vi "_Parse ES Flatness Limit Check Result.vi"(8 "error in (no error)":errorcluster, 10 "Input String":string, 11 "VISA resource name":refnum<visa-resource-name>) -> (0 "error out":errorcluster, 1 "Result":T1 {"Out Of Tolerance" format="%^.3e"}, 2 "Reliability":i32, 3 "VISA resource name out":refnum<visa-resource-name>)   [LabVIEW 2015, in "Rohde&Schwarz CMXP NR FR2 Measurement.lvlib"]
uses:
  <instrlib>/Rohde&Schwarz CMXP NR FR2 Measurement/Rohde&Schwarz CMXP NR FR2 Measurement.lvlib
  <instrlib>/Rohde&Schwarz CMXP NR FR2 Measurement/Private/rsidr_core.llb/rsidr_core.lvlib
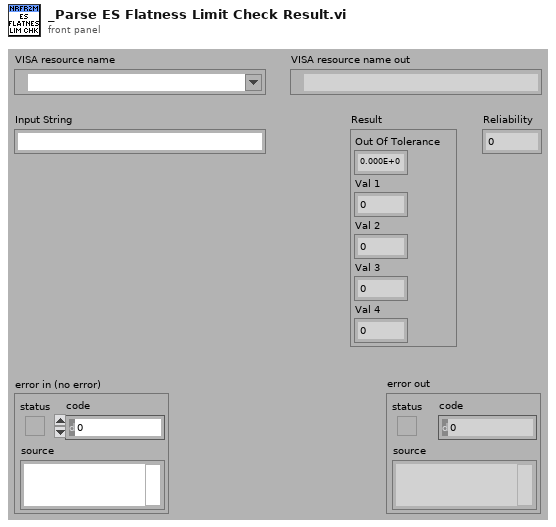
[diagram p1: front panel]
types:
  T1 = cluster{"Out Of Tolerance":dbl, "Val 1":i32, "Val 2":i32, "Val 3":i32, "Val 4":i32}
  T2 = cluster{"Out Of Tolerance":dbl, "Ripple 1":i32, "Ripple 2":i32, "Max R1 Min R2":i32, "Max R2 Min R1":i32}
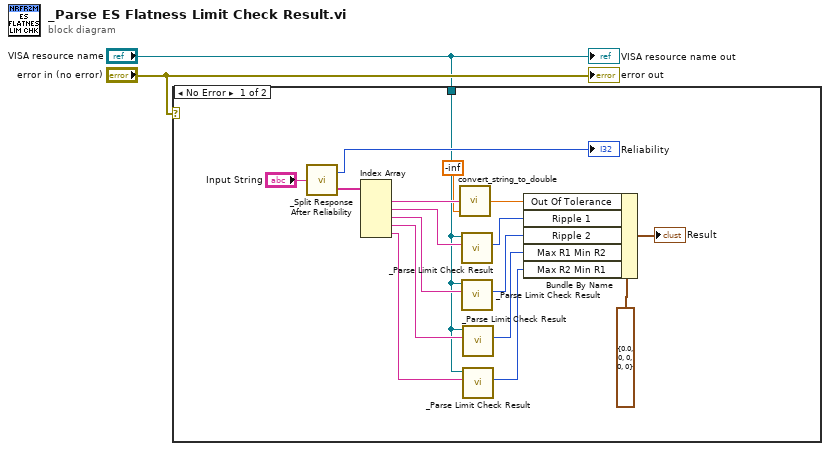
[diagram p0: block diagram]
diagram:
  n1 = case shown="No Error" "error in (no error)" {
    tunnel: "VISA resource name" -> [w3 _]
    frame No Error {
      n2 = call <instrlib>:"_Split Response After Reliability.vi"("Input String"="Input String") -> ("Response out"=w13:string[], "Reliability out"=→"Reliability":i32)
      n3 = Index Array(array=w13) -> (element #1=w12:string, element #2=w11:string, element #3=w10:string, element #4=w7:string, element #5=w8:string)  [unwired: 5 in]
      n4 = call <instrlib>:"convert_string_to_double.vi"("default (0)"=-inf, "String in"=w12) -> ("double value out"=w18:dbl)  [unwired: 3 in]
      n5 = call <instrlib>:"_Parse Limit Check Result.vi"("String Value In"=w11, "VISA resource name"=w3) -> ("Limit Check Value"=w17:i32)  [unwired: 7 in, 2 out]
      n6 = call <instrlib>:"_Parse Limit Check Result.vi"("String Value In"=w10, "VISA resource name"=w3) -> ("Limit Check Value"=w16:i32)  [unwired: 7 in, 2 out]
      n7 = call <instrlib>:"_Parse Limit Check Result.vi"("String Value In"=w7, "VISA resource name"=w3) -> ("Limit Check Value"=w5:i32)  [unwired: 7 in, 2 out]
      n8 = call <instrlib>:"_Parse Limit Check Result.vi"("String Value In"=w8, "VISA resource name"=w3) -> ("Limit Check Value"=w4:i32)  [unwired: 7 in, 2 out]
      n9 = Bundle By Name(cluster=T2 {"Out Of Tolerance"=0.0, "Ripple 1"=0, "Ripple 2"=0, "Max R1 Min R2"=0, "Max R2 Min R1"=0} ("Limit Check Result"), "Out Of Tolerance"=w18, "Ripple 1"=w17, "Ripple 2"=w16, "Max R1 Min R2"=w5, "Max R2 Min R1"=w4) -> (→"Result":T2)
    }
    frame Error {
    }
  }
  "VISA resource name out" <- "VISA resource name"
  "error out" <- "error in (no error)"
